vi "Send_Query_SCPI_Command.vi"(9 "Query Response?":bool, 10 "SCPI Command":string, 11 "VISA resource name":refnum<visa-resource-name>) -> ()   [LabVIEW 2025]
panel:
  out "error out":errorcluster
  in  "error in (no error)":errorcluster
  out "Response":string
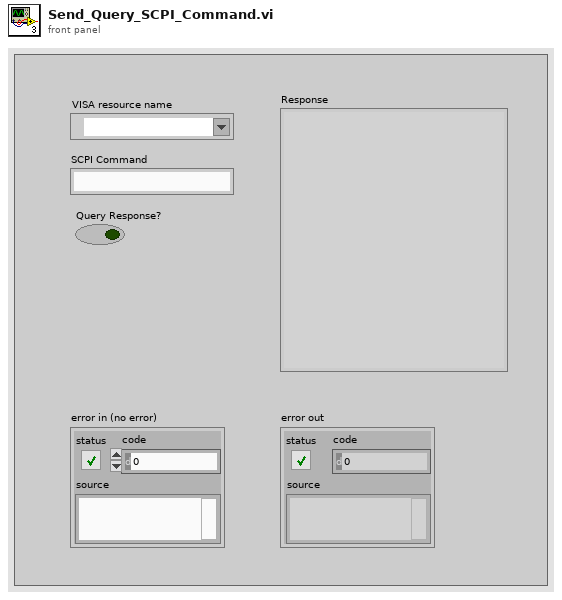
[diagram p1: front panel]
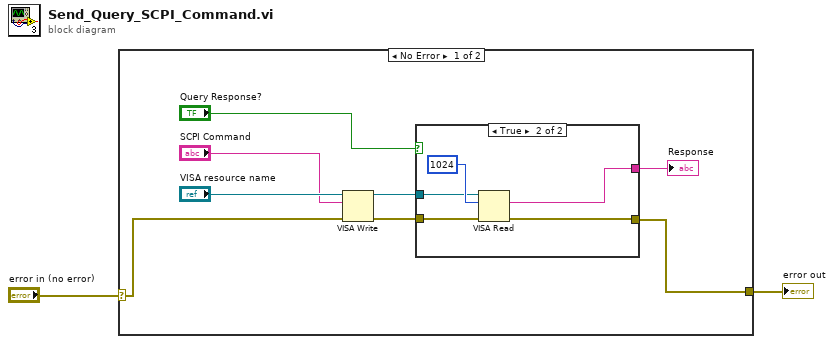
[diagram p0: block diagram]
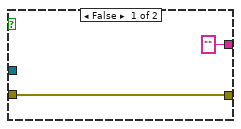
[diagram p2: hidden frame]
diagram:
  n1 = case shown="No Error" "error in (no error)" {
    selector: "error in (no error)" -> [w5 w18]
    tunnel: [w4 w18] -> w1
    frame No Error {
      n2 = VISA Write(VISA resource name="VISA resource name", write buffer="SCPI Command", error in (no error)=w5) -> (VISA resource name out=w7:refnum<visa-resource-name>, error out=w8:errorcluster)  [unwired: 1 out]
      n3 = case shown="True" "Query Response?" {
        tunnel: w8 -> [w12 w16]
        tunnel: w7 -> [_ w15]
        tunnel: [w12 w14] -> w4
        tunnel: ["" ("read buffer") w13] -> w3
        frame False {
        }
        frame True {
          n4 = VISA Read(VISA resource name=w15, byte count=u32 1024, error in (no error)=w16) -> (read buffer=w13:string, error out=w14:errorcluster)  [unwired: 2 out]
        }
      }
      "Response" <- w3
    }
    frame Error {
    }
  }
  "error out" <- w1
